vi "PH_Sequencer_Watch.PC calc Exp Vac State.vi"(0 "i ref in":refnum<vi>, 5 "error in":errorcluster) -> (14 "i ref out":refnum<vi>, 19 "error out":errorcluster)   [LabVIEW 2014, in "PH_Sequencer_Watch.lvlib"]
doc: "This VI indicates the status of the Exp Laserbay Vacuum State if it is of interest."
uses:
  PH_Sequencer_Watch.lvlib
  PH_Beamline_Chief/PH_Beamline_Chief.Section.ctl
  PH_Common/PH_Common.lvlib
  PH_BeamlineInformation/PH_BeamlineInformation.lvlib
  PH_Beamline_Chief/PH_Beamline_Chief.lvlib
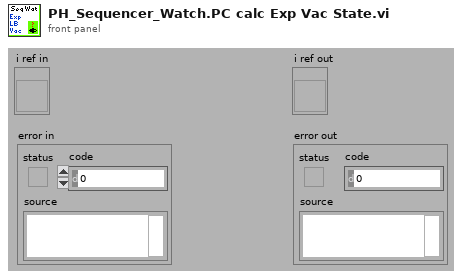
[diagram p1: front panel]
types:
  T1 = typedef "PH_Beamline_Chief.lvlib/PH_Beamline_Chief.Section.ctl" = enum16{"None", "YLF", "fs", "fs-YLF", "ns", "PA-Input", "PA-Undelay", "PA-Delay", "PA-before-Bypass", "PA", "PA-Bypass", "PA-Exit", "PA-LL", "LL", "PA-MA", "MA-Exit", "MA-Z6", "Z6", "MA-LB", "LB-TB2", "LB-TB3"}
  T2 = typedef "PH_Sequencer_Watch.lvlib/PH_Sequencer_Watch.i attribute.ctl" = cluster{"GUI Refs":cluster{"Shot ID":refnum<vi>, "Sequencer SM State":refnum<vi>, "Remaining Time":refnum<vi>, "PHELIX_Timing_T2":refnum<vi>, "T2-Unit-Dummy":refnum<vi>, "fs_Synchrolock_Watch":refnum<vi>, "Experiment_Vacuum_Control_Experiment":refnum<vi>}, "Status Synchrolock":T3, "Exp - Pressure":dbl, "Exp - Limit":dbl, "Heads":T4[], "Refs BooleanState":refnum<vi>[]}
  T3 = typedef "PH_StatusHandler.lvlib/PH_StatusHandler.Status.ctl" = i16
  T4 = typedef "PH_Sequencer_Watch.lvlib/PH_Sequencer_Watch.Head Information.ctl" = cluster{"Ref Volt":refnum<vi>, "PU":T5}
  T5 = typedef "PH_PP_Common.lvlib/PH_PP_Common.PUs.ctl" = enum16{"no Info", "PA-19mm-1", "PA-19mm-2", "PA-45mm-PILC", "PA-45mm-MAIN", "MA-PU-1", "MA-PU-2", "MA-PU-3", "MA-PU-4", "MA-PU-5", "MA-PU-6", "MA-FR", "MA-PILC", "PA-45mm-DP"}
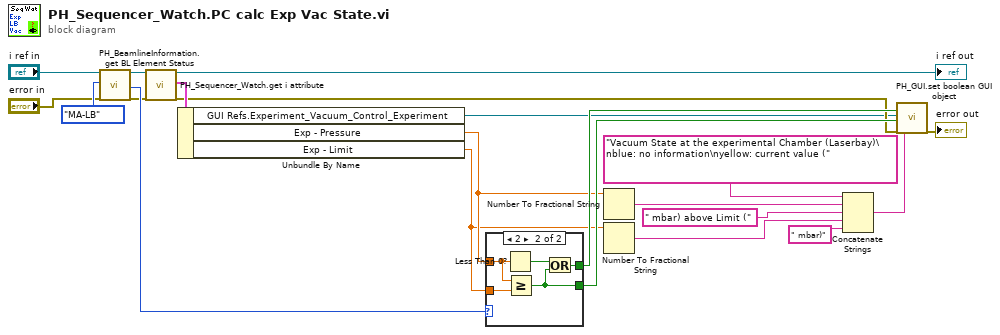
[diagram p0: block diagram]
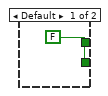
[diagram p2: hidden frame]
diagram:
  n1 = call "PH_BeamlineInformation.get BL Element Status.vi"("VI in"="i ref in", "Beamline Element"=PH_Beamline_Chief.Section."MA-LB", "error in (no error)"="error in") -> ("VI out"=w3:refnum<vi>, "Status"=w5:i32, "error out"=w2:errorcluster)  [unwired: 14 in]
  n2 = call "PH_Sequencer_Watch.get i attribute.vi"("i ref in"=w3, "error in (no error)"=w2) -> ("i ref out"=→"i ref out":refnum<vi>, "i attribute"=w21:T2, "error out"=w17:errorcluster)  [unwired: 15 in]
  n3 = Unbundle By Name(w21) -> ("GUI Refs.Experiment_Vacuum_Control_Experiment"=w15:refnum<vi>, "Exp - Pressure"=w12:dbl, "Exp - Limit"=w9:dbl)
  n4 = case shown="2" w5 {
    tunnel: w12 -> [_ w27]
    tunnel: [w22 w24] -> w20
    tunnel: [w22 w23] -> w19
    tunnel: w9 -> [_ w26]
    frame Default {
      w22 = FALSE
    }
    frame 2 {
      n5 = Less Than 0?(x=w27) -> (x < 0?=w25:bool)
      n6 = Greater Or Equal?(x=w27, y=w26) -> (x >= y?=w23:bool)
      n7 = Or(x=w25, y=w23) -> (x .or. y?=w24:bool)
    }
  }
  n8 = Number To Fractional String(number=w12) -> (F-format string=w11:string)  [unwired: 3 in]
  n9 = Number To Fractional String(number=w9) -> (F-format string=w8:string)  [unwired: 3 in]
  n10 = Concatenate Strings("Vacuum State at the experimental Chamber (Laserbay)\nblue: no information\nyellow: current value (" ("Tip Strip"), w11, " mbar) above Limit (" ("string"), w8, " mbar)" ("string")) -> (w13:string)
  n11 = call "PH_GUI.set boolean GUI object.vi"("Visible (true)"=w20, "Boolean Knob GUI Ref"=w15, "Value"=w19, "error in (no error)"=w17, "Tip Strip"=w13) -> ("error out"=→"error out":errorcluster)  [unwired: 14 in]
